vi "Old-RenameTIFFs_SIAMMetaDate.vi"(0 "folder path":path=path "\\\\till-server\\data/Entwicklung/PalmeMicrosystems/SIP-MicroSystems-Laser-20.11.2017/SIP-Chart-RawBilder") -> ()   [LabVIEW 2011]
panel:
  in  "testlauf":bool=TRUE
  out "result string":string="2017-11-20T163134.3101673"
  out "before substring":string="2017-11-20T16:31:34.3101673"
  out "string":string="<?xml version=\"1.0\" encoding=\"utf-8\"?>\r\n<OME xmlns:xsd=\"http://www.w3.org/2001/XMLSchema\" xmlns:xsi=\"http://www.w3.org/2001/XMLSchema-instance\" xsi:schemaLocation=\"http://www.openmicroscopy.org/Schemas/OME/2015-01 http://www.openmicroscopy.org/Schemas/OME/2015-01/ome.xsd\" UUID=\"urn:uuid:b3227219-734e-4715-b777-0266dcd872f5\" xmlns=\"http://www.openmicroscopy.org/Schemas/OME/2015-01\">\r\n  <Experiment ID=\"urn:lsid:till.id.de:Experiment:232ba7b5-e02d-450e-a87f-9f845788f511\">\r\n    <Description>ExperimentName: SIM_Slide_20.11.2017_16.24.01</Description>\r\n    <ExperimenterRef ID=\"urn:lsid:till.id.de:Experimenter:3dcd069a-fe4a-4674-8489-4e563baf8260\" />\r\n  </Experiment>\r\n  <Experimenter ID=\"urn:lsid:till.id.de:Experimenter:3dcd069a-fe4a-4674-8489-4e563baf8260\" UserName=\"Admin\" />\r\n  <Instrument ID=\"urn:lsid:till.id.de:Instrument:E61C7F75-E1FC-481B-859E-B66370AA4892\">\r\n    <Microscope Manufacturer=\"TILL I.D. GmbH\" Model=\"More\" />\r\n    <LightSource Model=\"EPI~System.Object\" ID=\"urn:lsid:till.id.de:LightSource:68a807fa-8c2e-40ba-a52c-cf6bed36c47a\">\r\n      <LightEmittingDiode />\r\n    </LightSource>\r\n    <LightSource Model=\"TRANS~System.Object\" ID=\"urn:lsid:till.id.de:LightSource:59ccea79-73d6-4cbe-b937-8329e8be0fa3\">\r\n      <LightEmittingDiode />\r\n    </LightSource>\r\n    <LightSource Model=\"SIM~ImageArena.Ome.OmeVersion201501.Laser\" ID=\"urn:lsid:till.id.de:LightSource:2e2a325e-bb76-43fd-87ef-f44117cae0a6\">\r\n      <Laser />\r\n    </LightSource>\r\n    <LightSource Model=\"TIRF~ImageArena.Ome.OmeVersion201501.Laser\" ID=\"urn:lsid:till.id.de:LightSource:71b667d8-45d4-4346-8232-22acf5148c0a\">\r\n      <Laser />\r\n    </LightSource>\r\n    <Detector Model=\"PCO_Edge4.2\" ID=\"urn:lsid:till.id.de:Detector:a52d56ec-a5c6-4f0a-80a4-0476bf18ffe4\" />\r\n    <Objective ID=\"urn:lsid:till.id.de:Objective:f2e891b1-aa2a-46bb-bad2-cf30486bfc63\" Immersion=\"Air\" LensNA=\"0.45\" NominalMagnification=\"10\" CalibratedMagnification=\"12.22\" />\r\n    <Objective ID=\"urn:lsid:till.id.de:Objective:aa165d83-0c1c-40a4-8a31-c8310ee6ae92\" Immersion=\"Air\" LensNA=\"0.8\" NominalMagnification=\"20\" CalibratedMagnification=\"24.44\" />\r\n    <Objective ID=\"urn:lsid:till.id.de:Objective:40839073-0823-4e4c-90a5-cc53fed433d1\" Immersion=\"Oil\" LensNA=\"1.4\" NominalMagnification=\"40\" CalibratedMagnification=\"48.52\" />\r\n    <Filter Model=\"Quad\" ID=\"urn:lsid:till.id.de:Filter:696c20fc-bd49-4db7-a8b5-c32693d7afd2\" />\r\n  </Instrument>\r\n  <Image ID=\"Image:bdbb100a-c6ed-43bd-8da3-f8159941b99a\">\r\n    <AcquisitionDate>2017-11-20T16:31:34.3101673+01:00</AcquisitionDate>\r\n    <InstrumentRef ID=\"urn:lsid:till.id.de:Instrument:E61C7F75-E1FC-481B-859E-B66370AA4892\" />\r\n    <ObjectiveSettings ID=\"urn:lsid:till.id.de:Objective:f2e891b1-aa2a-46bb-bad2-cf30486bfc63\" />\r\n    <Pixels ID=\"Pixels:0\" DimensionOrder=\"XYZTC\" Type=\"uint16\" SizeX=\"2048\" SizeY=\"1024\" SizeZ=\"11\" SizeC=\"1\" SizeT=\"1\" PhysicalSizeX=\"0.5319149\" PhysicalSizeY=\"0.5319149\" PhysicalSizeZ=\"2\">\r\n      <Channel ID=\"Channel:0:-1\" SamplesPerPixel=\"1\" IlluminationType=\"Other\" AcquisitionMode=\"StructuredIllumination\" EmissionWavelength=\"561\">\r\n        <DetectorSettings ID=\"urn:lsid:till.id.de:Detector:a52d56ec-a5c6-4f0a-80a4-0476bf18ffe4\" />\r\n        <LightPath />\r\n      </Channel>\r\n      <TiffData IFD=\"0\" FirstZ=\"0\" FirstT=\"0\" FirstC=\"0\" PlaneCount=\"11\">\r\n        <UUID FileName=\"77_SIM0_561nm.tif\">urn:uuid:b3227219-734e-4715-b777-0266dcd872f5</UUID>\r\n      </TiffData>\r\n      <Plane TheZ=\"0\" TheT=\"0\" TheC=\"0\" DeltaT=\"0\" PositionX=\"-4940.94727\" PositionXUnit=\"µm\" PositionY=\"1880.972\" PositionYUnit=\"µm\" PositionZ=\"6740\" PositionZUnit=\"µm\" />\r\n      <Plane TheZ=\"1\" TheT=\"0\" TheC=\"0\" DeltaT=\"0.3797976\" PositionX=\"-4940.94727\" PositionXUnit=\"µm\" PositionY=\"1880.972\" PositionYUnit=\"µm\" PositionZ=\"6742\" PositionZUnit=\"µm\" />\r\n      <Plane TheZ=\"2\" TheT=\"0\" TheC=\"0\" DeltaT=\"0.7600472\" PositionX=\"-4940.94727\" PositionXUnit=\"µm\" PositionY=\"1880.972\" PositionYUnit=\"µm\" PositionZ=\"6744\" PositionZUnit=\"µm\" />\r\n      <Plane TheZ=\"3\" TheT=\"0\" TheC=\"0\" DeltaT=\"1.14217281\" PositionX=\"-4940.94727\" PositionXUnit=\"µm\" PositionY=\"1880.972\" PositionYUnit=\"µm\" PositionZ=\"6746\" PositionZUnit=\"µm\" />\r\n      <Plane TheZ=\"4\" TheT=\"0\" TheC=\"0\" DeltaT=\"1.520685\" PositionX=\"-4940.94727\" PositionXUnit=\"µm\" PositionY=\"1880.972\" PositionYUnit=\"µm\" PositionZ=\"6748\" PositionZUnit=\"µm\" />\r\n      <Plane TheZ=\"5\" TheT=\"0\" TheC=\"0\" DeltaT=\"1.90025413\" PositionX=\"-4940.94727\" PositionXUnit=\"µm\" PositionY=\"1880.972\" PositionYUnit=\"µm\" PositionZ=\"6750\" PositionZUnit=\"µm\" />\r\n      <Plane TheZ=\"6\" TheT=\"0\" TheC=\"0\" DeltaT=\"2.280702\" PositionX=\"-4940.94727\" PositionXUnit=\"µm\" PositionY=\"1880.972\" PositionYUnit=\"µm\" PositionZ=\"6752\" PositionZUnit=\"µm\" />\r\n      <Plane TheZ=\"7\" TheT=\"0\" TheC=\"0\" DeltaT=\"2.66071272\" PositionX=\"-4940.94727\" PositionXUnit=\"µm\" PositionY=\"1880.972\" PositionYUnit=\"µm\" PositionZ=\"6754\" PositionZUnit=\"µm\" />\r\n      <Plane TheZ=\"8\" TheT=\"0\" TheC=\"0\" DeltaT=\"3.040997\" PositionX=\"-4940.94727\" PositionXUnit=\"µm\" PositionY=\"1880.972\" PositionYUnit=\"µm\" PositionZ=\"6756\" PositionZUnit=\"µm\" />\r\n      <Plane TheZ=\"9\" TheT=\"0\" TheC=\"0\" DeltaT=\"3.4203558\" PositionX=\"-4940.94727\" PositionXUnit=\"µm\" PositionY=\"1880.972\" PositionYUnit=\"µm\" PositionZ=\"6758\" PositionZUnit=\"µm\" />\r\n      <Plane TheZ=\"10\" TheT=\"0\" TheC=\"0\" DeltaT=\"3.80167341\" PositionX=\"-4940.94727\" PositionXUnit=\"µm\" PositionY=\"1880.972\" PositionYUnit=\"µm\" PositionZ=\"6760\" PositionZUnit=\"µm\" />\r\n    </Pixels>\r\n  </Image>\r\n  <StructuredAnnotations xmlns=\"http://www.openmicroscopy.org/Schemas/SA/2015-01\">\r\n    <XMLAnnotation ID=\"Annotation:0\" Namespace=\"http://www.openmicroscopy.org/omero/dimension/modulo\">\r\n      <Value>\r\n        <Modulo xmlns=\"http://www.openmicroscopy.org/Schemas/Addition/2015-01\" xmlns:OME=\"http://www.openmicroscopy.org/Schemas/OME/2015-01\">\r\n          <ModuloAlongT Type=\"tile\" Start=\"0\" End=\"0\" Step=\"1\" xmlns=\"\" />\r\n        </Modulo>\r\n      </Value>\r\n    </XMLAnnotation>\r\n  </StructuredAnnotations>\r\n</OME>"
  out "Input-File":i32=3
  out "Files":path[](array[path])=[path "\\\\till-server\\data/Entwicklung/PalmeMicrosystems/SIP-MicroSystems-Laser-20.11.2017/SIP-Chart-RawBilder/70_ZStack_SIM0_561nm_d7b9489b-8507-41b8-905d-3407818c6e7d/70_SIM0_561nm.tif", path "\\\\till-server\\data/Entwicklung/PalmeMicrosystems/SIP-MicroSystems-Laser-20.11.2017/SIP-Chart-RawBilder/72_ZStack_SIM0_561nm_0e398477-0201-4661-9848-fb1709e88dee/72_SIM0_561nm.tif", path "\\\\till-server\\data/Entwicklung/PalmeMicrosystems/SIP-MicroSystems-Laser-20.11.2017/SIP-Chart-RawBilder/75_ZStack_SIM0_561nm_6d9a4cf7-7532-4e4a-b69c-7ef8fb9b2cf6/75_SIM0_561nm.tif", path "\\\\till-server\\data/Entwicklung/PalmeMicrosystems/SIP-MicroSystems-Laser-20.11.2017/SIP-Chart-RawBilder/77_ZStack_SIM0_561nm_bdbb100a-c6ed-43bd-8da3-f8159941b99a/77_SIM0_561nm.tif"]
  # "select folder\nfirst tiff in subfolder will be renamed with Aqusition date!\ncreated 2016 who need this now?"
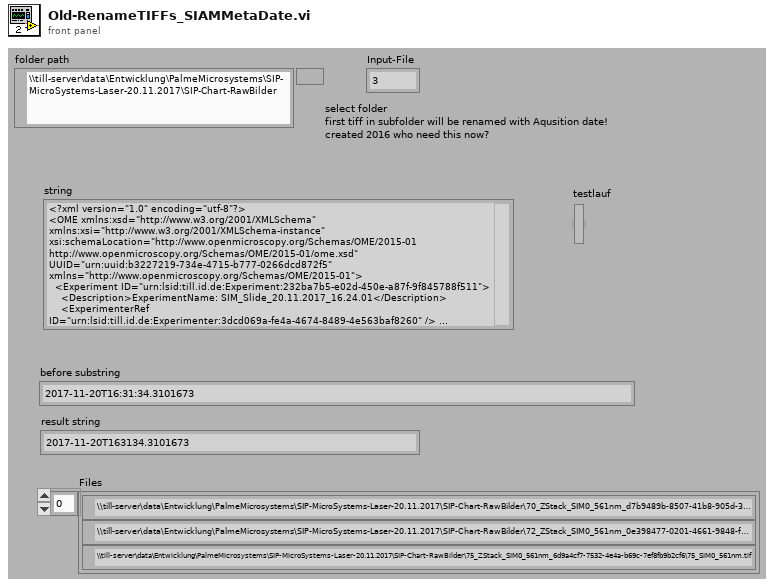
[diagram p1: front panel]
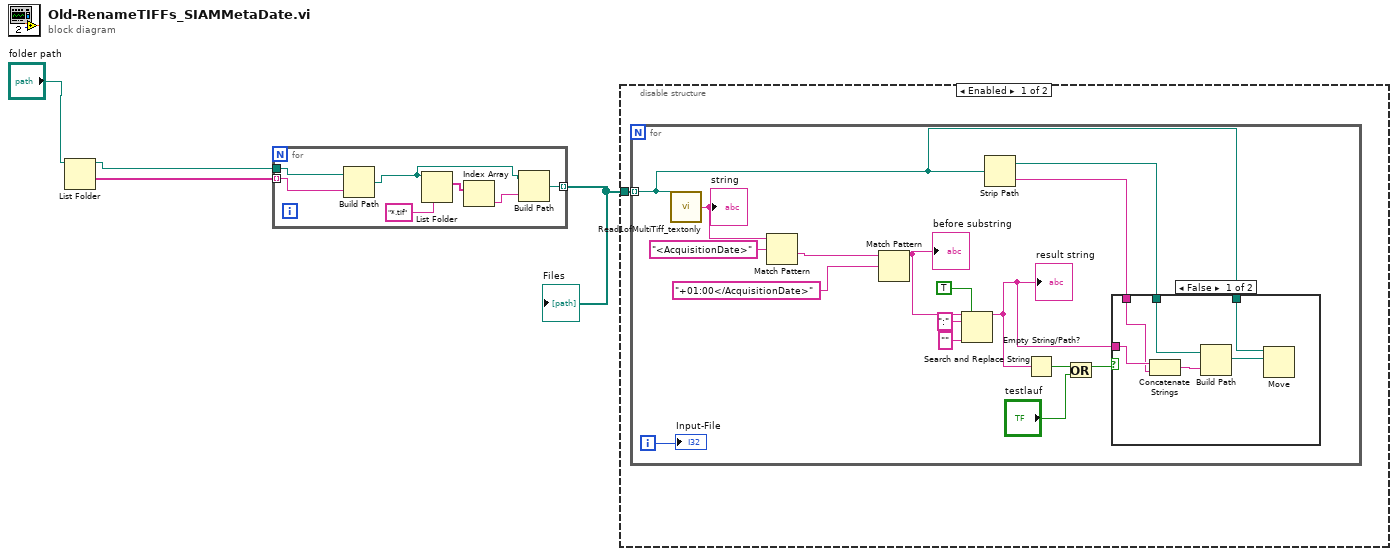
[diagram p0: block diagram]
diagram:
  n1 = List Folder(path="folder path") -> (path out=w1:path, folder names=w2:string[])  [unwired: 3 in, 2 out]
  n2 = for {
    tunnel: [w11] -> w4 mode=indexing
    tunnel: w2 -> [w6] mode=indexing
    tunnel: w1 -> [w7]
    n3 = Build Path(base path=w7, name or relative path=w6) -> (appended path=w5:path)
    n4 = List Folder(path=w5, pattern="*.tif") -> (filenames=w9:string[])  [unwired: 2 in, 3 out]
    n5 = Index Array(array=w9) -> (element=w8:string)  [unwired: 1 in]
    n6 = Build Path(base path=w5, name or relative path=w8) -> (appended path=w11:path)
  }
  "Files" <- w4
  n7 = disable-structure shown="Enabled" {
    disable-tunnel: w4 -> [w12 _]
    frame Enabled {
      n8 = for {
        tunnel: w12 -> [w15] mode=indexing
        i -> [w28]
        n9 = call "Read1ofMultiTiff_textonly.vi"("file path"=w15) -> ("string"=w27:string)  [unwired: 3 in, 1 out]
        "string" <- w27
        n10 = Match Pattern(string=w27, regular expression="<AcquisitionDate>") -> (after substring=w25:string)  [unwired: 1 in, 3 out]
        n11 = Match Pattern(string=w25, regular expression="+01:00</AcquisitionDate>") -> (before substring=w23:string)  [unwired: 1 in, 3 out]
        "before substring" <- w23
        n12 = Search and Replace String(replace all?=TRUE ("replace all? (F)"), input string=w23, search string=":", replace string="" ("replace string (\"\")")) -> (result string=w18:string)  [unwired: 4 in, 3 out]
        "result string" <- w18
        n13 = Strip Path(path=w15) -> (stripped path=w17:path, name=w16:string)
        n14 = Empty String/Path?(string/path=w18) -> (empty?=w19:bool)
        n15 = Or(x=w19, y="testlauf") -> (x .or. y?=w14:bool)
        n16 = case shown="False" w14 {
          tunnel: w18 -> [w33 _]
          tunnel: w17 -> [w34 _]
          tunnel: w16 -> [w32 _]
          tunnel: w15 -> [w30 _]
          frame False {
            n17 = Concatenate Strings(w33, w32) -> (w31:string)
            n18 = Build Path(base path=w34, name or relative path=w31) -> (appended path=w29:path)
            n19 = Move(source path=w30, 10:w29) -> ()  [unwired: 3 in, 3 out]
          }
          frame True {
          }
        }
        "Input-File" <- w28
      }
    }
    frame Disabled {
    }
  }
